vi "Interpret Force From Raw Data.vi"   [LabVIEW 2013]
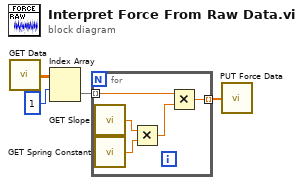
[diagram p0: block diagram]
diagram:
  n1 = call "GET Data.vi"() -> ("Data"=w3:dbl[][])
  n2 = Index Array(array=w3, index (row)=1) -> (element=w2:dbl[])  [unwired: 1 in]
  n3 = for {
    tunnel: [w9] -> w1 mode=indexing
    tunnel: w2 -> [w5] mode=indexing
    n4 = call "GET Slope.vi"() -> ("Slope"=w7:dbl)
    n5 = call "GET Spring Constant.vi"() -> ("Spring Constant"=w6:dbl)
    n6 = Multiply(x=w7, y=w6) -> (x*y=w8:dbl)
    n7 = Multiply(x=w5, y=w8) -> (x*y=w9:dbl)
  }
  n8 = call "PUT Force Data.vi"("Force Data"=w1) -> ()
